vi "Create All Message Queues.vi"(8 "error in (no error)":errorcluster {"code" format="Error %.0f"}) -> (0 "error out":errorcluster {"code" format="Error %.0f"}, 3 "messageQueuesOut":T1)   [LabVIEW 2017, in "Message Queue.lvlib"]
doc: "This VI creates and initializes all the message queues for your application. If your application requires more than one message queue, right-click the \"Message Queues\" constant above and select Open Type Def. Add the new Message Queue(s) to the type definition, then initialize them in this VI."
uses:
  Message Queue.lvlib
  messageQueues.ctl
  Message Cluster.ctl
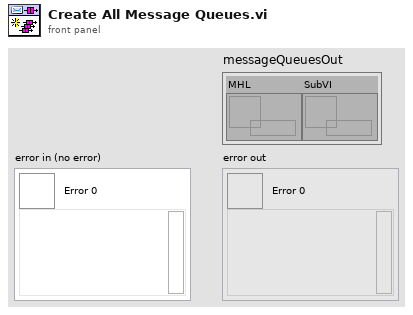
[diagram p1: front panel]
types:
  T1 = typedef "Message Queue.lvlib/messageQueues.ctl" = cluster{"MHL":refnum<queue>, "SubVI":refnum<queue>}
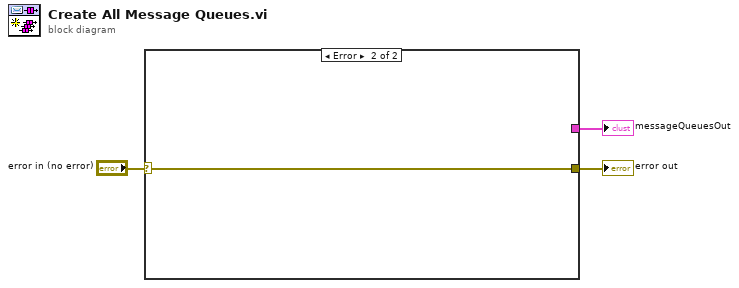
[diagram p0: block diagram]
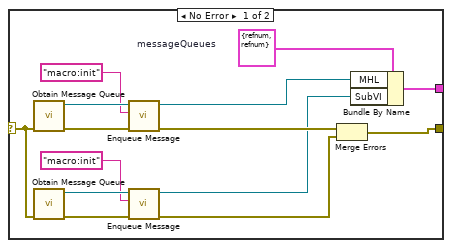
[diagram p2: hidden frame]
diagram:
  n1 = case shown="Error" "error in (no error)" {
    selector: "error in (no error)" -> [w10 w18]
    tunnel: [w15 w18] -> w1
    tunnel: [w16 _] -> w3
    frame No Error {
      w17 = T1 {"MHL"=refnum, "SubVI"=refnum}  # messageQueues
      n2 = call "Obtain Message Queue.vi"("error in (no error)"=w10) -> ("error out"=w14:errorcluster, "Message Queue"=w12:refnum<queue>)  [unwired: 9 in]
      n3 = call "Obtain Message Queue.vi"("error in (no error)"=w10) -> ("error out"=w8:errorcluster, "Message Queue"=w9:refnum<queue>)  [unwired: 9 in]
      n4 = call "Enqueue Message.vi"("error in (no error)"=w14, "Message"="macro:init", "Message Queue"=w12) -> ("error out"=w13:errorcluster, "dup Message Queue"=w11:refnum<queue>)  [unwired: 7 in]
      n5 = call "Enqueue Message.vi"("error in (no error)"=w8, "Message"="macro:init", "Message Queue"=w9) -> ("error out"=w7:errorcluster, "dup Message Queue"=w4:refnum<queue>)  [unwired: 7 in]
      n6 = Merge Errors(w13, w7) -> (w15:errorcluster)
      n7 = Bundle By Name(cluster=w17, "MHL"=w11, "SubVI"=w4) -> (w16:T1)
    }
    frame Error {
    }
  }
  "messageQueuesOut" <- w3
  "error out" <- w1
